vi "无效产品.vi"() -> ()   [LabVIEW 2020]
uses:
  System.Windows.Forms
panel:
  in  "ToolStrip":refnum<k24>(container)
  # "当前选择的产品型号有误\n请检查产品型号是否符合规范"
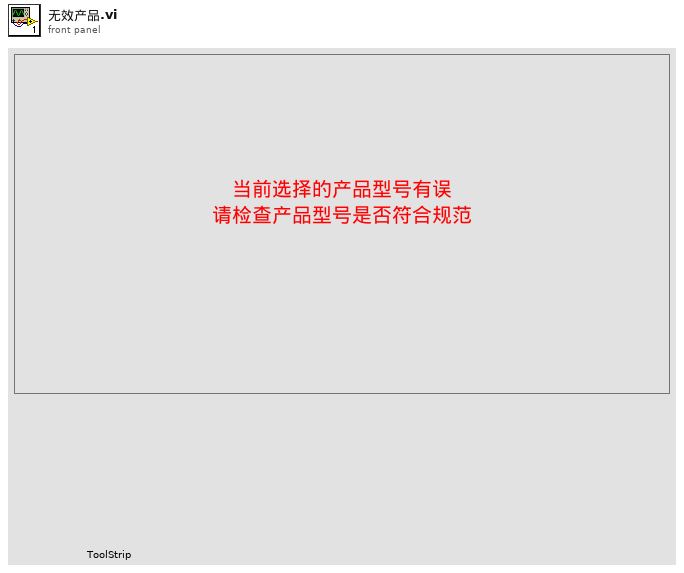
[diagram p1: front panel]
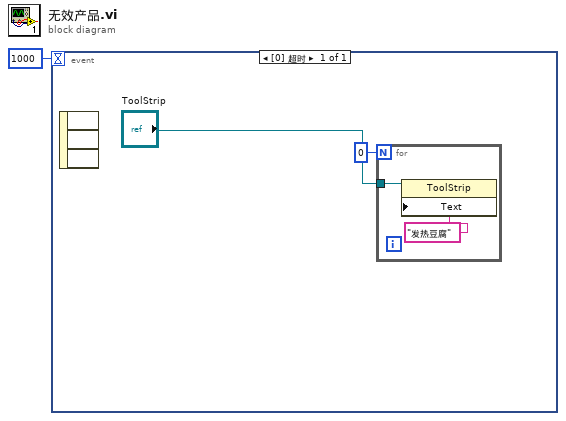
[diagram p0: block diagram]
diagram:
  n1 = event shown="[0] 超时" {
    selector: _ -> [_]
    dyn-events: _ -> [_]
    timeout: 1000 -> [_]
    event Timeout {
      n2 = event-data() -> ()  [unwired: 1 in, 3 out]
      n3 = for {
        N: 0 -> [_]
        tunnel: "ToolStrip" -> [w5]
        n4 = property class="ToolStrip"(reference=w5, "Text"="发热豆腐" ("ToString")) -> ()  [unwired: 1 in, 2 out]
      }
    }
  }
